vi "arbitraryMiniScan.vi"(9 "Norm zStop in":dbl, 10 "Norm zStart":dbl, 11 "FrameSize":i32) -> (1 "StepSize":dbl, 2 "min_coordinate":dbl)   [LabVIEW 2017]
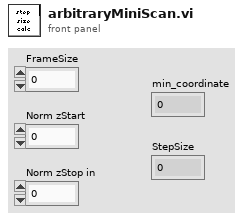
[diagram p1: front panel]
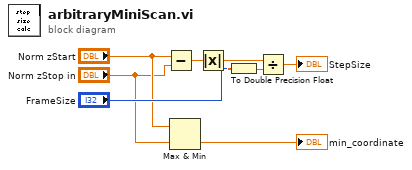
[diagram p0: block diagram]
diagram:
  n1 = Subtract(x="Norm zStart", y="Norm zStop in") -> (x-y=w6:dbl)
  n2 = Max & Min(x="Norm zStart", y="Norm zStop in") -> (min(x,y)=→"min_coordinate":dbl)  [unwired: 1 out]
  n3 = Absolute Value(x=w6) -> (abs(x)=w5:dbl)
  n4 = To Double Precision Float(number="FrameSize") -> (double precision float=w7:dbl)
  n5 = Divide(x=w5, y=w7) -> (x/y=→"StepSize":dbl)
